vi "SampleDetails.vi"(0 "NewSample in Obs":bool, 1 "SampleGoal":string, 2 "SampleDetailsClus":T1) -> (3 "SampleName":string, 4 "SampleNameNoDate":string)   [LabVIEW 2019]
panel:
  out "date/time string":string
  out "resulting string":string
  out "Synthesis/Polymer":string
  out "String":string
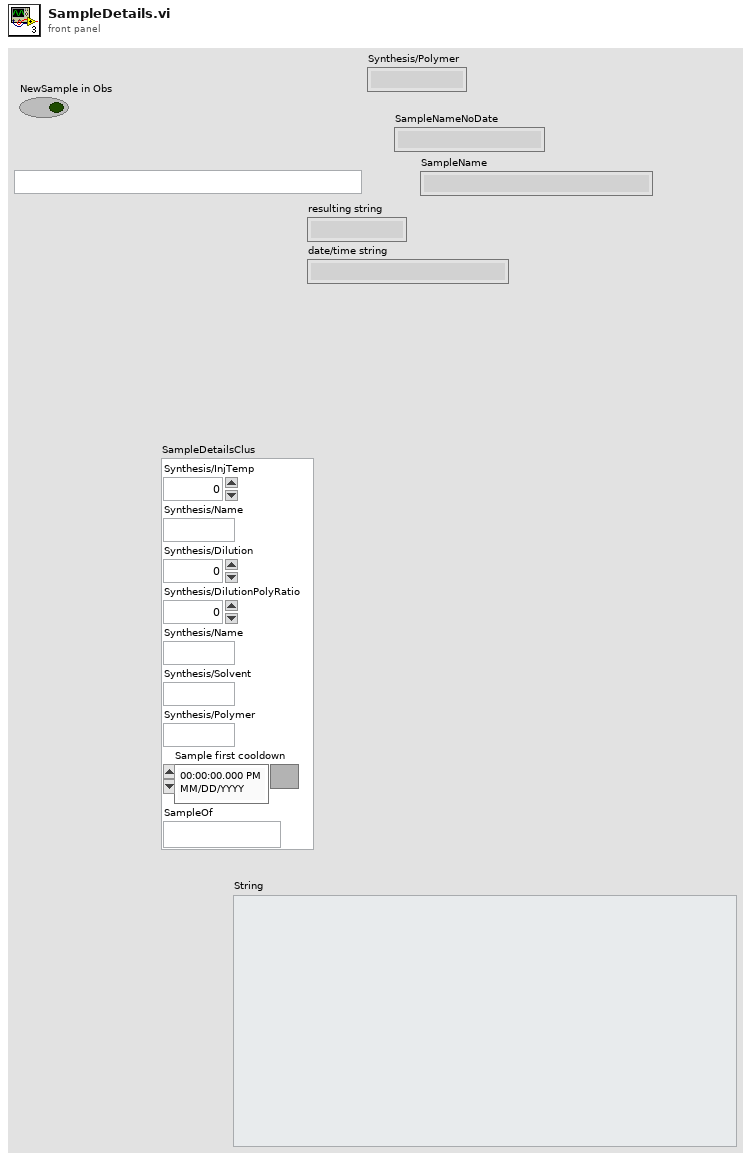
[diagram p1: front panel]
types:
  T1 = cluster{"Synthesis/InjTemp":dbl, "Synthesis/Name":string, "Synthesis/Dilution":dbl, "Synthesis/DilutionPolyRatio":dbl, "Synthesis/Name":string, "Synthesis/Solvent":string, "Synthesis/Polymer":string, "Sample first cooldown":timestamp, "SampleOf":string}
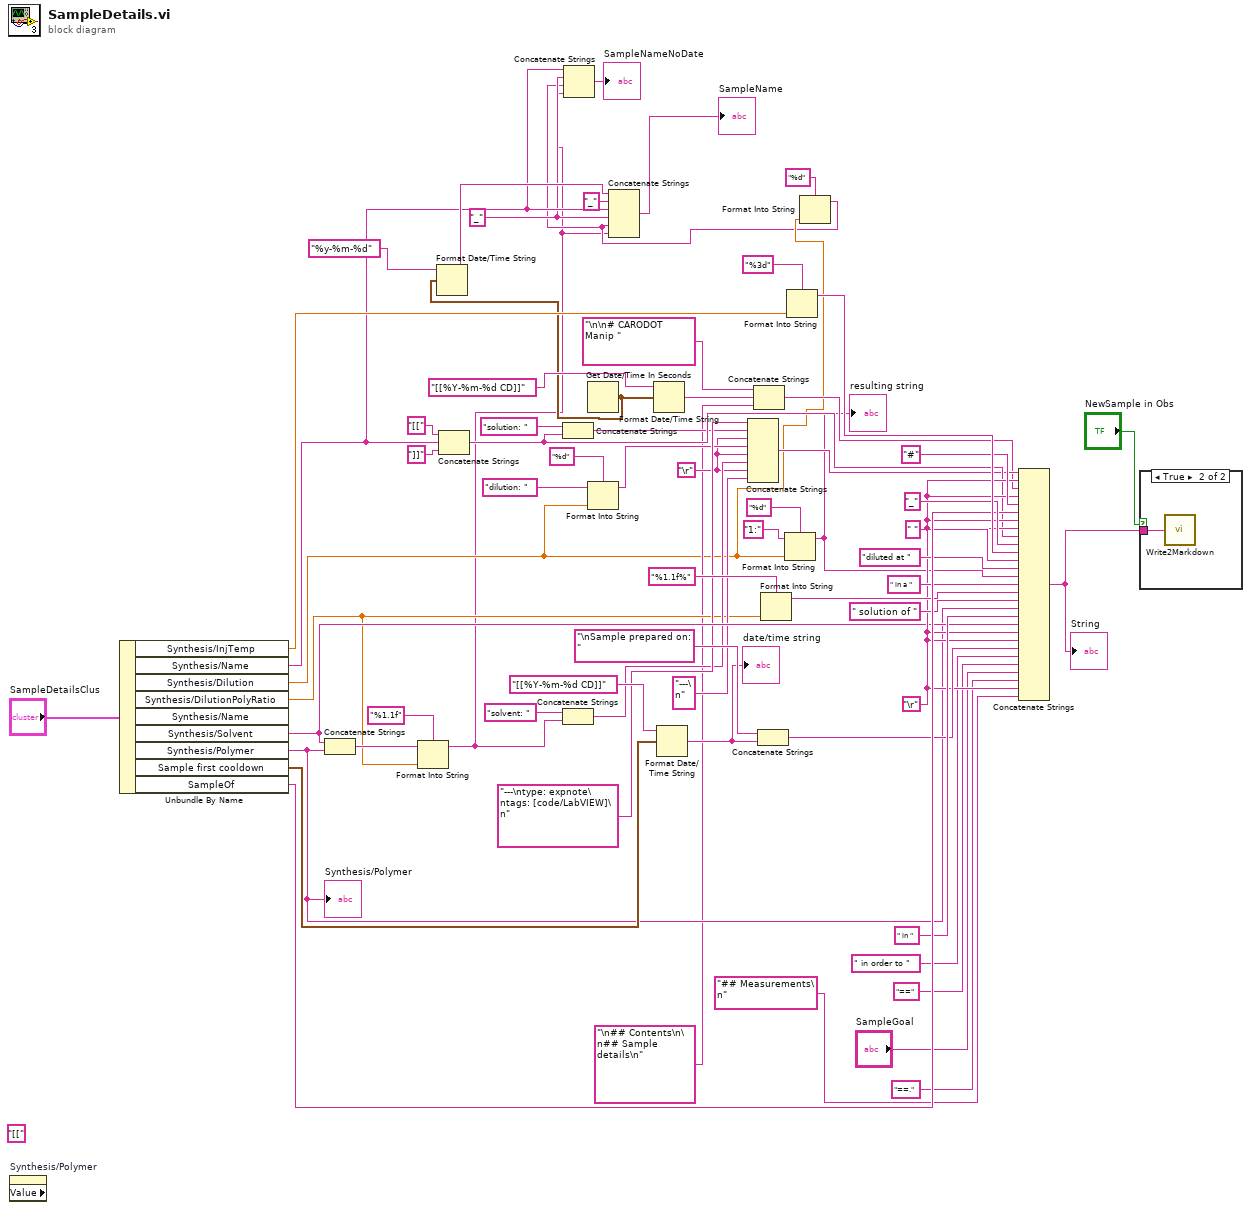
[diagram p0: block diagram]
diagram:
  w5 = "_" ("string")
  (unwired) "[[" ("string")
  w27 = "\r"
  w42 = "\r"
  n1 = property on="Synthesis/Polymer" class="Str" props=["Value"]() -> ()  [unwired: 2 in, 3 out]
  n2 = Unbundle By Name("SampleDetailsClus") -> ("Synthesis/InjTemp"=w65:dbl, "Synthesis/Name"=w6:string, "Synthesis/Dilution"=w7:dbl, "Synthesis/DilutionPolyRatio"=w24:dbl, "Synthesis/Solvent"=w36:string, "Synthesis/Polymer"=w35:string, "Sample first cooldown"=w50:timestamp, "SampleOf"=w60:string)  [unwired: 1 out]
  "Synthesis/Polymer" <- w35
  n3 = Concatenate Strings(w36, w35) -> (w33:string)
  n4 = Format Into String(format string="%1.1f", initial string=w33, w24) -> (resulting string=w3:string)  [unwired: 1 in, 1 out]
  n5 = Concatenate Strings("[[", w6, "]]") -> (w39:string)
  n6 = Concatenate Strings("solution: ", w39) -> (w30:string)
  n7 = Concatenate Strings("solvent: ", w3) -> (w28:string)
  n8 = Get Date/Time In Seconds() -> (seconds since 1Jan1904=w13:timestamp)
  n9 = Format Date/Time String(time format string (%c)="%y-%m-%d", seconds (now)=w13) -> (date/time string=w11:string)  [unwired: 1 in]
  n10 = Format Into String(format string="%d", initial string="dilution: ", w7) -> (resulting string=w29:string)  [unwired: 1 in, 1 out]
  n11 = Format Date/Time String(time format string (%c)="[[%Y-%m-%d CD]]", seconds (now)=w13) -> (date/time string=w20:string)  [unwired: 1 in]
  n12 = Format Date/Time String(time format string (%c)="[[%Y-%m-%d CD]]", seconds (now)=w50) -> (date/time string=w47:string)  [unwired: 1 in]
  "date/time string" <- w47
  n13 = Concatenate Strings("---\ntype: expnote\ntags: [code/LabVIEW]\n", w30, w27, w29, w27, w28, w27, "---\n" ("string")) -> (w25:string)
  n14 = Concatenate Strings("\n\n# CARODOT Manip ", w20, "\n## Contents\n\n## Sample details\n" ("string")) -> (w23:string)
  n15 = Concatenate Strings("\nSample prepared on: " ("string"), w47) -> (w46:string)
  n16 = Format Into String(format string="%1.1f%", w24) -> (resulting string=w57:string)  [unwired: 2 in, 1 out]
  n17 = Format Into String(format string="%d", initial string="1:", w7) -> (resulting string=w9:string)  [unwired: 1 in, 1 out]
  "resulting string" <- w9
  n18 = Format Into String(format string="%3d", w65) -> (resulting string=w64:string)  [unwired: 2 in, 1 out]
  n19 = Format Into String(format string="%d", w7) -> (resulting string=w4:string)  [unwired: 2 in, 1 out]
  n20 = Concatenate Strings(w6, w5, w4, w3) -> (→"SampleNameNoDate":string)
  n21 = Concatenate Strings(w11, "_" ("string"), w6, w5, w4, w3) -> (→"SampleName":string)
  n22 = Concatenate Strings(w25, w42, w23, w42, "#" ("string"), w60, w42, w42, w39, "_" ("string"), w64, " " ("string"), "diluted at " ("string"), w9, " in a " ("string"), w57, " solution of " ("string"), w35, " in " ("string"), w36, w42, w42, w46, " in order to " ("string"), "==" ("string"), "SampleGoal", "==." ("string"), w42, "## Measurements\n") -> (w43:string)
  "String" <- w43
  n23 = case shown="True" "NewSample in Obs" {
    tunnel: w43 -> [_ w67]
    frame False {
    }
    frame True {
      n24 = call "Write2Markdown.vi"("String"=w67) -> ()
    }
  }
